vi "read comm response.vi"(8 "error in (no error)":errorcluster, 11 "Roda_Filtros in":refnum<class "Roda_Filtros.lvclass">) -> (0 "error out":errorcluster, 3 "Roda_Filtros out":refnum<class "Roda_Filtros.lvclass">)   [LabVIEW 2018, in "Roda_Filtros.lvclass"]
uses:
  Roda_Filtros.lvclass
  Roda_Filtros.lvclass/Roda_Filtros.ctl
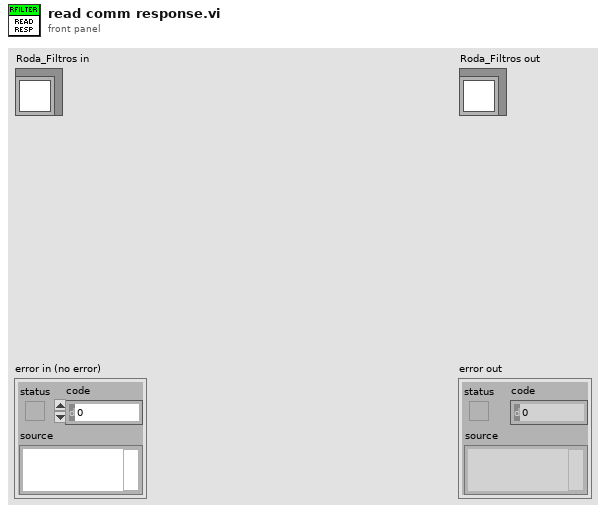
[diagram p1: front panel]
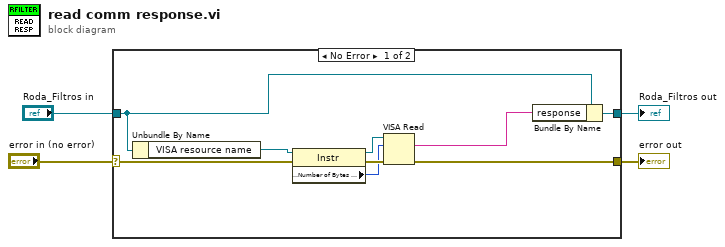
[diagram p0: block diagram]
diagram:
  n1 = case shown="No Error" "error in (no error)" {
    selector: "error in (no error)" -> [w12 w15]
    tunnel: [w11 w15] -> w3
    tunnel: [w10 w14] -> w1
    tunnel: "Roda_Filtros in" -> [w8 w14]
    frame No Error {
      n2 = Unbundle By Name(w8) -> ("VISA resource name"=w13:refnum<visa-resource-name>)
      n3 = property class="Instr"(reference=w13, error in=w12) -> (reference out=w7:refnum<visa-resource-name>, error out=w6:errorcluster, "Serial Settings:Number of Bytes at Serial Port"=w5:u32)
      n4 = VISA Read(VISA resource name=w7, byte count=w5, error in (no error)=w6) -> (read buffer=w9:string, error out=w11:errorcluster)  [unwired: 2 out]
      n5 = Bundle By Name(cluster=w8, "response"=w9) -> (w10:refnum<class "Roda_Filtros.lvclass">)
    }
    frame Error {
    }
  }
  "error out" <- w3
  "Roda_Filtros out" <- w1
